vi "New Result.vi"(8 "error in (no error)":errorcluster, 9 "parameter":string, 10 "function":string, 11 "id":string) -> (0 "error out":errorcluster, 3 "result":refnum<class "result.lvclass">)   [LabVIEW 2015, in "result.lvclass"]
uses:
  result.lvclass
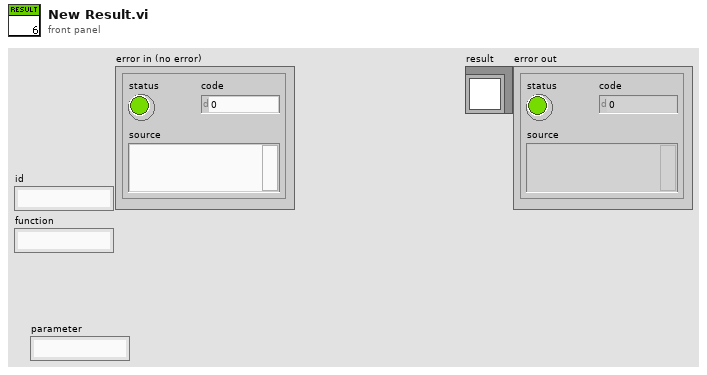
[diagram p1: front panel]
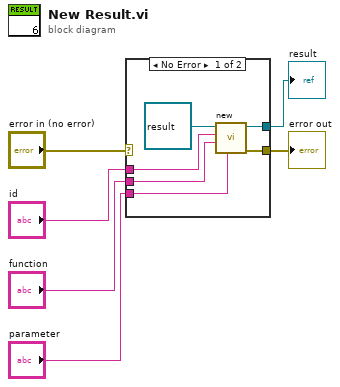
[diagram p0: block diagram]
diagram:
  n1 = case shown="No Error" "error in (no error)" {
    selector: "error in (no error)" -> [_ w13]
    tunnel: "id" -> [w11 _]
    tunnel: "function" -> [w10 _]
    tunnel: [w7 _] -> w4
    tunnel: "parameter" -> [w9 _]
    tunnel: [w8 w13] -> w1
    frame No Error {
      n2 = call "new.vi"("parameter"=w9, "function"=w10, "id"=w11, "result"=refnum<class "result.lvclass"> refnum ("result.lvclass")) -> ("error Out"=w8:errorcluster, "result"=w7:refnum<class "result.lvclass">)  [unwired: 6 in]
    }
    frame Error {
    }
  }
  "result" <- w4
  "error out" <- w1
